vi "MuC_Parse_Read.vi"(1 "Buffer Data":string[](array[string])) -> (0 "Data":dbl[][](array[numeric]))   [LabVIEW 2019]
doc: "Parse the readings from the read buffer into an array of numerical values\n\nR. Sheehan 28 - 10 - 2020"
panel:
  out "Nreads":i32
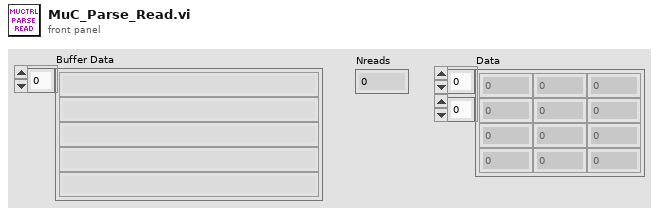
[diagram p1: front panel]
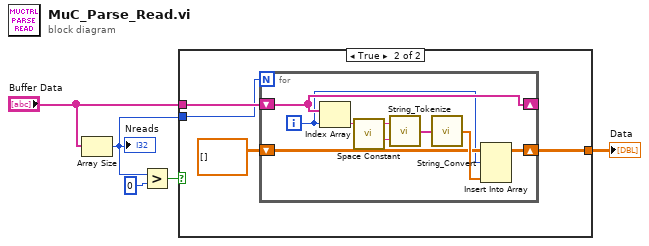
[diagram p0: block diagram]
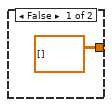
[diagram p2: hidden frame]
diagram:
  n1 = Array Size(array="Buffer Data") -> (size(s)=w3:i32)
  "Nreads" <- w3
  n2 = Greater?(x=w3, y=0) -> (0:w1:bool)
  n3 = case shown="True" w1 {
    tunnel: "Buffer Data" -> [_ w10]
    tunnel: [dbl[][] [] w8] -> w4
    tunnel: w3 -> [_ w7]
    frame False {
    }
    frame True {
      n4 = for {
        N: w7 -> [_]
        shift-right: [w17] -> _
        shift-left: w10 -> [w17]
        shift-right: [w12] -> w8
        shift-left: dbl[][] [] -> [w13]
        i -> [w11]
        n5 = Index Array(array=w17, index=w11) -> (element=w16:string)
        n6 = call <vilib>:"Space Constant.vi"() -> ("String"=w18:string)
        n7 = call "String_Tokenize.vi"("String Token"=w18, "String"=w16) -> ("String Array"=w15:string[])
        n8 = call "String_Convert.vi"("String Array"=w15) -> ("Numerical Array"=w14:dbl[])
        n9 = Insert Into Array(array=w13, index (row)=w11, new element=w14) -> (w12:dbl[][])  [unwired: 1 in]
      }
    }
  }
  "Data" <- w4
